vi "ProtoBuff - Decode Array of Bytes.vi"(10 "Encoded String":string="\\370\\360\\005\\244\\247\\301") -> (1 "Array of Bytes":u8[](array[numeric]), 2 "Hexidecimal Strings":string[](array[string]))   [LabVIEW 2020]
doc: "Decodes an array of bytes, encoded as a numeric string by protobuf."
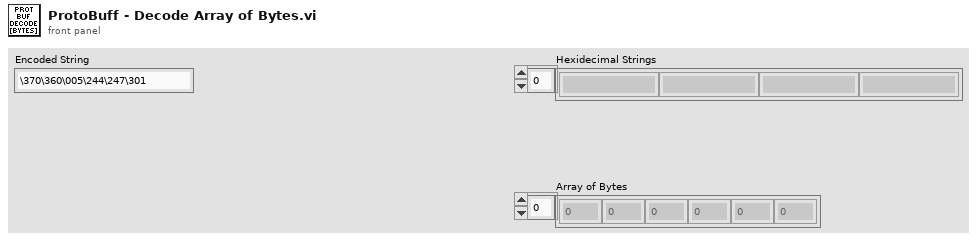
[diagram p1: front panel]
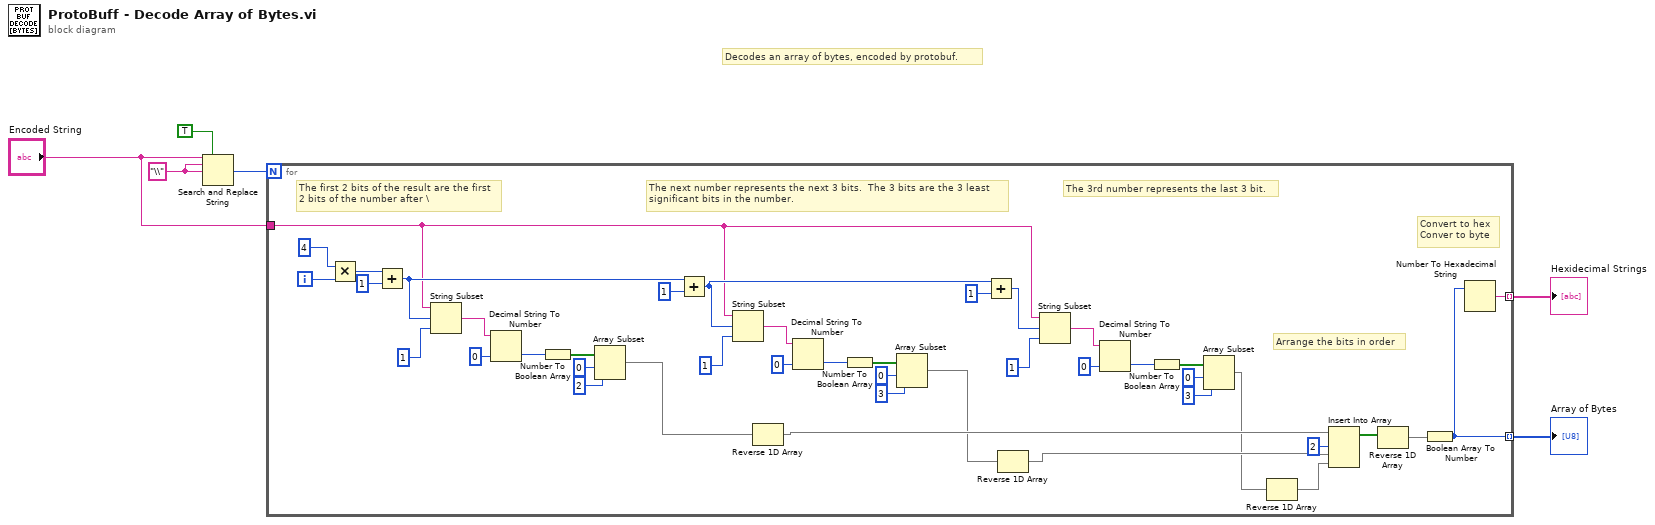
[diagram p0: block diagram]
diagram:
  w6 = "\\" ("search string")
  # "Decodes an array of bytes, encoded by protobuf."
  n1 = Search and Replace String(replace all?=TRUE ("replace all? (F)"), input string="Encoded String", search string=w6, replace string=w6) -> (number of replacements=w5:i32)  [unwired: 4 in, 3 out]
  n2 = for {
    N: w5 -> [_]
    tunnel: "Encoded String" -> [w18]
    tunnel: [w8] -> w2 mode=indexing
    tunnel: [w7] -> w1 mode=indexing
    i -> [w46]
    # "Convert to hex\nConver to byte"
    # "Arrange the bits in order"
    # "The 3rd number represents the last 3 bit."
    # "The next number represents the next 3 bits.  The 3 bits are the 3 least\nsignificant bits in the number."
    # "The first 2 bits of the result are the first\n2 bits of the number after \\"
    n3 = Multiply(x=4, y=w46) -> (x*y=w44:i32)
    n4 = Add(x=w44, y=1) -> (x+y=w29:i32)
    n5 = String Subset(string=w18, offset (0)=w29, length (rest)=1 ("length (rest)")) -> (substring=w41:string)
    n6 = Decimal String To Number(string=w41, default (0L)=u8 0 ("default (0 I32)")) -> (number=w48:u8)  [unwired: 1 in, 1 out]
    n7 = Number To Boolean Array(number=w48) -> (Boolean array=w40:bool[])
    n8 = Array Subset(array=w40, index=0, length=2) -> (w16:bool[])
    n9 = Add(x=w29, y=1) -> (x+y=w19:i32)
    n10 = String Subset(string=w18, offset (0)=w19, length (rest)=1 ("length (rest)")) -> (substring=w33:string)
    n11 = Reverse 1D Array(array=w16) -> (reversed array=w15:bool[])
    n12 = Decimal String To Number(string=w33, default (0L)=u8 0 ("default (0 I32)")) -> (number=w37:u8)  [unwired: 1 in, 1 out]
    n13 = Number To Boolean Array(number=w37) -> (Boolean array=w32:bool[])
    n14 = Array Subset(array=w32, index=0, length=3) -> (w14:bool[])
    n15 = Add(x=w19, y=1) -> (x+y=w25:i32)
    n16 = Reverse 1D Array(array=w14) -> (reversed array=w13:bool[])
    n17 = String Subset(string=w18, offset (0)=w25, length (rest)=1 ("length (rest)")) -> (substring=w23:string)
    n18 = Decimal String To Number(string=w23, default (0L)=u8 0 ("default (0 I32)")) -> (number=w28:u8)  [unwired: 1 in, 1 out]
    n19 = Number To Boolean Array(number=w28) -> (Boolean array=w22:bool[])
    n20 = Array Subset(array=w22, index=0, length=3) -> (w12:bool[])
    n21 = Reverse 1D Array(array=w12) -> (reversed array=w11:bool[])
    n22 = Insert Into Array(array=w15, index=2, new element #1=w13, new element #2=w11) -> (w10:bool[])
    n23 = Reverse 1D Array(array=w10) -> (reversed array=w9:bool[])
    n24 = Boolean Array To Number(Boolean array=w9) -> (number=w8:u32)
    n25 = Number To Hexadecimal String(2:w8) -> (0:w7:string)  [unwired: 1 in]
  }
  "Array of Bytes" <- w2
  "Hexidecimal Strings" <- w1
